vi "Read Event References.vi"(8 "error in (no error)":errorcluster, 11 "serenial.io-ase in":refnum<class "ase.lvclass">) -> (0 "error out":errorcluster, 2 "Event References":T1, 3 "serenial.io-ase out":refnum<class "ase.lvclass">)   [LabVIEW 2020, in "serenial.io-ase.lvlib" / "ase.lvclass"]
doc: "Read the User Event References."
uses:
  ase.lvclass
  Event References.ctl
  Standard Output.ctl
  Standard Error.ctl
  Did Exit.ctl
  ase.lvclass/ase.ctl
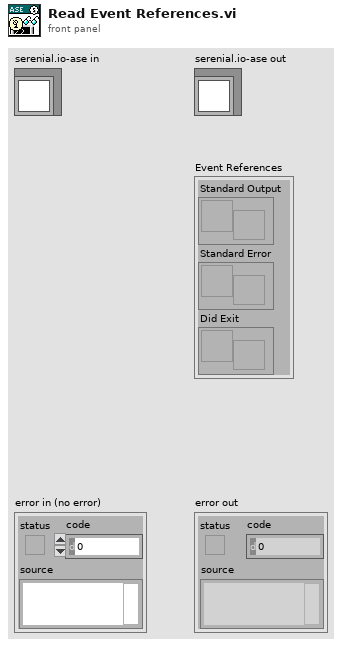
[diagram p1: front panel]
types:
  T1 = typedef "serenial.io-ase.lvlib/ase.lvclass/Event References.ctl" = cluster{"Standard Output":refnum<user-event>, "Standard Error":refnum<user-event>, "Did Exit":refnum<user-event>}
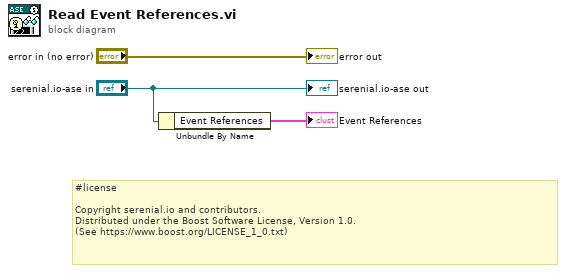
[diagram p0: block diagram]
diagram:
  # "#license\n\nCopyright serenial.io and contributors.\nDistributed under the Boost Software License, Version 1.0.\n(See https://www.boost.org/LICENSE_1_0.txt)"
  n1 = Unbundle By Name("serenial.io-ase in") -> ("Event References"=→"Event References":T1)
  "error out" <- "error in (no error)"
  "serenial.io-ase out" <- "serenial.io-ase in"
